vi "Time_Since_Threshold.vi"(1 "Mode":T1, 2 "History Length (mins)":dbl=1.0, 3 "Threshold Valve":dbl=0.5, 4 "Channel Name":string="GMU:Source:Divertor Valve") -> (0 "Time Greater than (s)":dbl)   [LabVIEW 2022 SP3]
uses:
  Sub VIs/Threshold_Mode.ctl
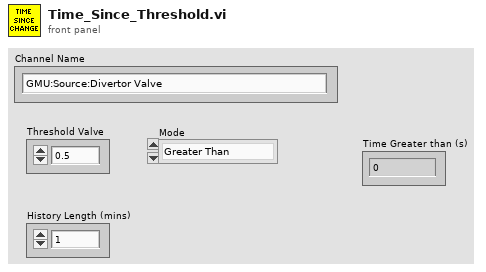
[diagram p1: front panel]
types:
  T1 = typedef "Threshold_Mode.ctl" = enum16{"Greater Than", "Less Than"}
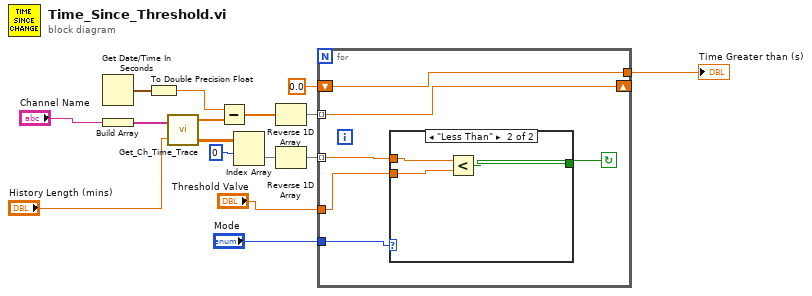
[diagram p0: block diagram]
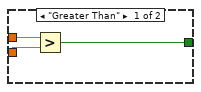
[diagram p2: hidden frame]
diagram:
  n1 = Get Date/Time In Seconds() -> (seconds since 1Jan1904=w15:timestamp)
  n2 = Build Array("Channel Name") -> (w16:string[])
  n3 = To Double Precision Float(number=w15) -> (double precision float=w14:dbl)
  n4 = call "Get_Ch_Time_Trace.vi"("Desired Ch Names"=w16, "History Length (mins)"="History Length (mins)") -> ("Centre Times"=w13:dbl[], "Output array"=w12:dbl[][])  [unwired: 1 out]
  n5 = Subtract(x=w14, y=w13) -> (x-y=w10:dbl[])
  n6 = Index Array(array=w12, index (row)=0) -> (element=w9:dbl[])  [unwired: 1 in]
  n7 = Reverse 1D Array(array=w10) -> (reversed array=w7:dbl[])
  n8 = Reverse 1D Array(array=w9) -> (reversed array=w8:dbl[])
  n9 = for {
    tunnel: w8 -> [w22] mode=indexing
    tunnel: w7 -> [w20] mode=indexing
    shift-right: [w20] -> _
    shift-left: 0.0 -> [w19]
    tunnel: [w19] -> w5
    tunnel: "Threshold Valve" -> [w18]
    tunnel: "Mode" -> [w17]
    stop <- w21 continue-if-true
    n10 = case shown="\"Less Than\"" w17 {
      tunnel: w22 -> [w25 w28]
      tunnel: [w24 w26] -> w21
      tunnel: w18 -> [w23 w27]
      frame "Greater Than" {
        n11 = Greater?(x=w25, y=w23) -> (0:w24:bool)
      }
      frame "Less Than" {
        n12 = Less?(x=w28, y=w27) -> (x < y?=w26:bool)
      }
    }
  }
  "Time Greater than (s)" <- w5
